vi "CylinderLayerGen.vi"(6 "Layer":u32=160, 10 "HatchPow":T6={"Power"=300.0, "Mark Speed"=400.0, "Jump Speed"=1000.0}, 11 "CircHatch":T1={"Diameter"=1.0, "Angle"=45.0, "Offset"=0.1, "Spacing"=0.1} {"Spacing" format="%#_13g"; "Offset" format="%#_13g"; "Diameter" format="%#_13g"}) -> (3 "PathSups":T2[](array[typedef]))   [LabVIEW 2014]
uses:
  TypeDefs/PowerSpeed.ctl
  TypeDefs/PathSupreme.ctl
  PSup2SCAN/Sub/VelocityProfile.ctl
  PSup2SCAN/Sub/PathCut.ctl
  PSup2SCAN/Sub/Segment.ctl
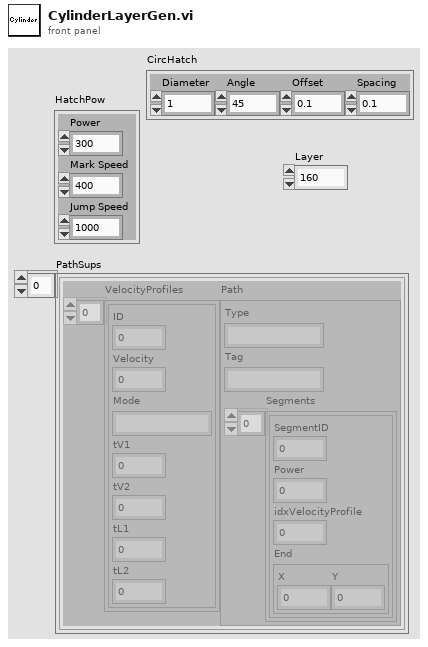
[diagram p1: front panel]
types:
  T1 = cluster{"Diameter":dbl, "Angle":sgl, "Offset":dbl, "Spacing":dbl}
  T2 = typedef "PathSupreme.ctl" = cluster{"VelocityProfiles":T3[], "Path":T4}
  T3 = typedef "VelocityProfile.ctl" = cluster{"ID":u32, "Velocity":dbl, "Mode":string, "tV1":u32, "tV2":u32, "tL1":u32, "tL2":u32}
  T4 = typedef "PathCut.ctl" = cluster{"Type":string, "Tag":string, "Segments":T5[]}
  T5 = typedef "Segment.ctl" = cluster{"SegmentID":u16, "Power":sgl, "idxVelocityProfile":u16, "End":cluster{"X":sgl, "Y":sgl}}
  T6 = typedef "PowerSpeed.ctl" = cluster{"Power":dbl, "Mark Speed":dbl, "Jump Speed":dbl}
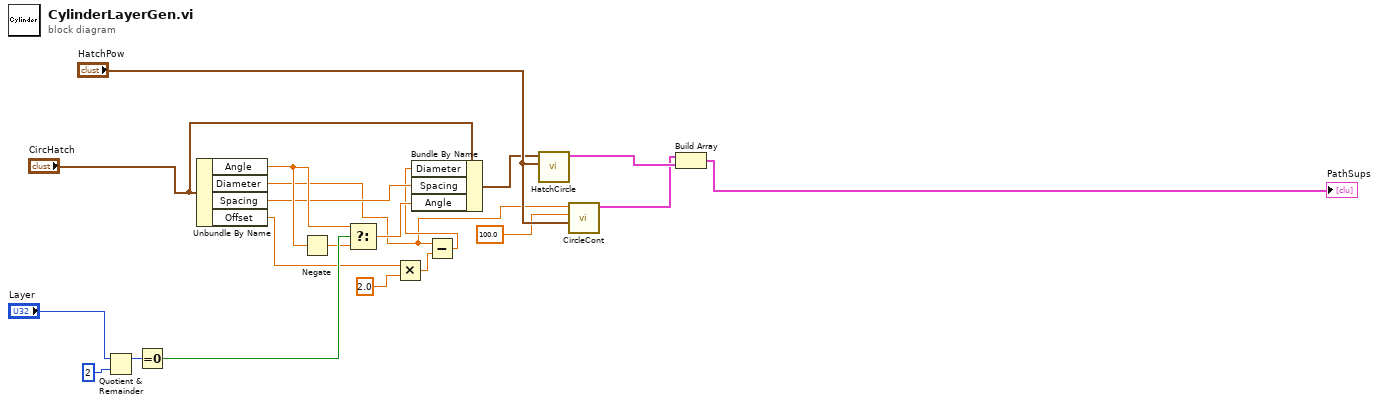
[diagram p0: block diagram]
diagram:
  n1 = Quotient & Remainder(x="Layer", y=u8 2) -> (x-y*floor(x/y)=w20:u32)  [unwired: 1 out]
  n2 = Equal To 0?(x=w20) -> (x = 0?=w17:bool)
  n3 = Unbundle By Name("CircHatch") -> ("Angle"=w13:sgl, "Diameter"=w1:dbl, "Spacing"=w10:dbl, "Offset"=w6:dbl)
  n4 = Negate(x=w13) -> (-x=w14:sgl)
  n5 = Select(t=w13, s=w17, f=w14) -> (s? t:f=w12:sgl)
  n6 = Multiply(x=w6, y=2.0) -> (x*y=w5:dbl)
  n7 = Subtract(x=w1, y=w5) -> (x-y=w2:dbl)
  n8 = Bundle By Name(cluster="CircHatch", "Diameter"=w2, "Spacing"=w10, "Angle"=w12) -> (w11:T1)
  n9 = call "HatchCircle.vi"("HatchPow"="HatchPow", "CircHatch"=w11) -> ("PathSupreme"=w9:T2)  [unwired: 9 in]
  n10 = call "CircleCont.vi"("ContPow"="HatchPow", "NumSides"=100.0, "Diameter"=w1) -> ("PathSupreme"=w3:T2)  [unwired: 8 in]
  n11 = Build Array(w3, w9) -> (→"PathSups":T2[])
